vi "TCD.vi"(6 "limitTheta2":dbl=100.0, 7 "limitTheta1":dbl=100.0, 8 "L2":dbl, 9 "L1":dbl, 10 "theta2":dbl, 11 "theta1":dbl) -> (1 "py":dbl, 2 "px":dbl)   [LabVIEW 2019]
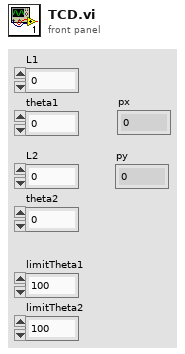
[diagram p1: front panel]
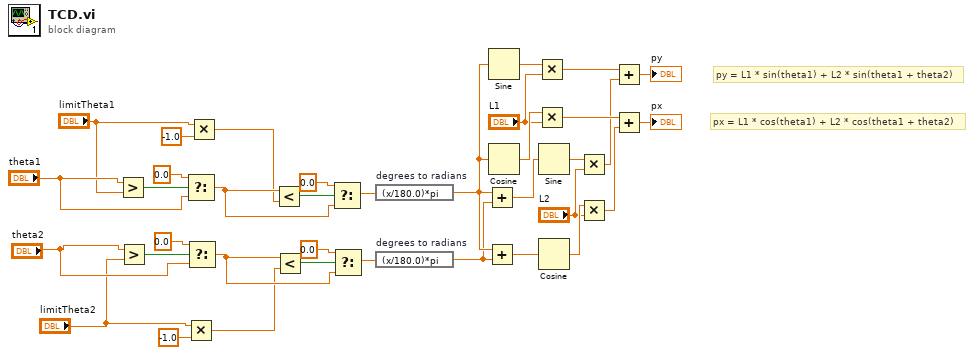
[diagram p0: block diagram]
diagram:
  # "py = L1 * sin(theta1) + L2 * sin(theta1 + theta2)"
  # "px = L1 * cos(theta1) + L2 * cos(theta1 + theta2)"
  n1 = Greater?(x="theta1", y="limitTheta1") -> (0:w16:bool)
  n2 = Greater?(x="theta2", y="limitTheta2") -> (0:w11:bool)
  n3 = Select(t=0.0, s=w16, f="theta1") -> (s? t:f=w18:dbl)
  n4 = Multiply(x="limitTheta2", y=-1.0) -> (x*y=w1:dbl)
  n5 = Select(t=0.0, s=w11, f="theta2") -> (s? t:f=w13:dbl)
  n6 = Multiply(x="limitTheta1", y=-1.0) -> (x*y=w3:dbl)
  n7 = Less?(x=w18, y=w3) -> (x < y?=w17:bool)
  n8 = Less?(x=w13, y=w1) -> (x < y?=w12:bool)
  n9 = Select(t=0.0, s=w17, f=w18) -> (s? t:f=w10:dbl)
  n10 = Select(t=0.0, s=w12, f=w13) -> (s? t:f=w8:dbl)
  n11 = expression code="(x/180.0)*pi" "degrees to radians"(w10) -> (w23:dbl)
  n12 = expression code="(x/180.0)*pi" "degrees to radians"(w8) -> (w22:dbl)
  n13 = Add(x=w23, y=w22) -> (x+y=w26:dbl)
  n14 = Add(x=w23, y=w22) -> (x+y=w32:dbl)
  n15 = Sine(x=w23) -> (sin(x)=w31:dbl)
  n16 = Cosine(x=w23) -> (cos(x)=w36:dbl)
  n17 = Multiply(x=w31, y="L1") -> (x*y=w30:dbl)
  n18 = Multiply(x=w36, y="L1") -> (x*y=w35:dbl)
  n19 = Sine(x=w26) -> (sin(x)=w29:dbl)
  n20 = Cosine(x=w32) -> (cos(x)=w34:dbl)
  n21 = Multiply(x=w29, y="L2") -> (x*y=w28:dbl)
  n22 = Multiply(x=w34, y="L2") -> (x*y=w21:dbl)
  n23 = Add(x=w30, y=w28) -> (x+y=→"py":dbl)
  n24 = Add(x=w35, y=w21) -> (x+y=→"px":dbl)
